vi "Broadcast New Layout.vi"(8 "error in (no error)":errorcluster, 9 "Pixel <> Zone":T1, 10 "Cage Diagram ref":T2) -> (0 "error out":errorcluster)   [LabVIEW 2018, in "Cage Diagram.lvlib"]
doc: "Broadcasts new layout and array of pixel to zone correspondences.\n_____\nCreated using Delacor QMH Event Scripter 4.2.1.88."
uses:
  Cage Diagram.lvlib
  <vilib>/vision/Image Controls.llb/IMAQ Image.ctl
  SubVi's/Controls/CTL_Pixel_to_Zone_array.ctl
  Broadcast New Layout Argument--cluster.ctl
  Common_Resources.lvlib
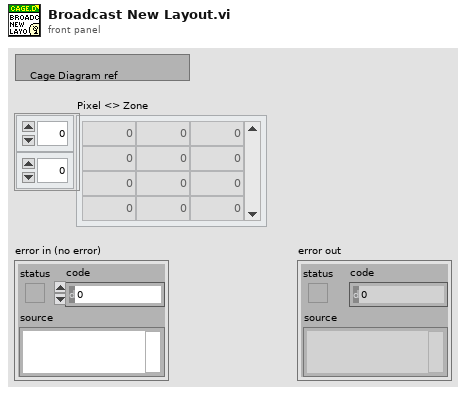
[diagram p1: front panel]
types:
  T1 = typedef "Common_Resources.lvlib/CTL_Pixel_to_Zone_array.ctl" = i8[][]
  T2 = typedef "IMAQ Image.ctl" = refnum<image>
  T3 = typedef "Cage Diagram.lvlib/Broadcast New Layout Argument--cluster.ctl" = cluster{"Cage Diagram ref":T2, "Pixel <> Zone":T1}
  T4 = typedef "Cage Diagram.lvlib/Broadcast Events--cluster.ctl" = cluster{"Module Did Init":refnum<user-event>, "Status Updated":refnum<user-event>, "Error Reported":refnum<user-event>, "Module Did Stop":refnum<user-event>, "Update Module Execution Status":refnum<user-event>, "Broadcast New Layout":refnum<user-event>}
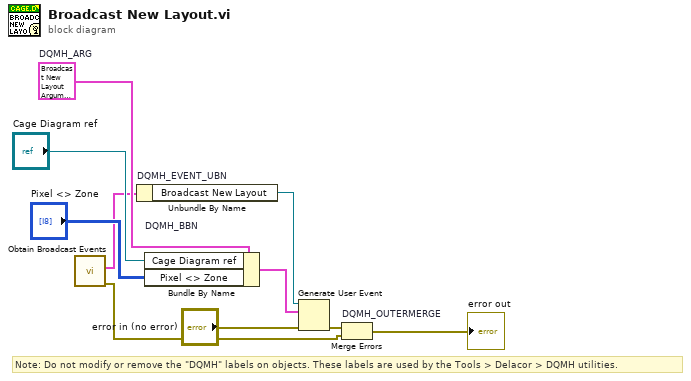
[diagram p0: block diagram]
diagram:
  w5 = T3 {"Cage Diagram ref"=refnum, "Pixel <> Zone"=[]}  # DQMH_ARG
  # "Note: Do not modify or remove the \"DQMH\" labels on objects. These labels are used by the Tools > Delacor > DQMH utilities."
  n1 = call "Obtain Broadcast Events.vi"() -> ("error out"=w2:errorcluster, "Cage Diagram Broadcast Events"=w1:T4)  [unwired: 10 in]
  n2 = Unbundle By Name "DQMH_EVENT_UBN"(w1) -> ("Broadcast New Layout"=w7:refnum<user-event>)
  n3 = Bundle By Name "DQMH_BBN"(cluster=w5, "Cage Diagram ref"="Cage Diagram ref", "Pixel <> Zone"="Pixel <> Zone") -> (w8:T3)
  n4 = Generate User Event(user event=w7, event data cluster=w8, error in="error in (no error)") -> (error out=w6:errorcluster)  [unwired: 1 in, 1 out]
  n5 = Merge Errors "DQMH_OUTERMERGE"(w6, w2) -> (→"error out":errorcluster)
